vi "Kinect_Data_Detection.vi"(0 "KinectSensor References in":T1, 5 "Image":T2, 7 "Distance from Kinect (m)":dbl=1.03 format="%#_13g", 11 "error in (no error)":errorcluster) -> (1 "X (m)":dbl format="%#.2f", 2 "Y (m)":dbl format="%#.2f", 3 "Z (m)":dbl format="%#.2f", 4 "KinectSensor References":T1, 6 "Image Out":T2, 8 "Distance from Kinect (calibrated, m)":dbl, 15 "Error Out":errorcluster)   [LabVIEW 2015]
uses:
  <vilib>/MakerHub/KinectOne/Private/Type Defs/KinectSensor References.ctl
  Microsoft.Kinect
  C:/Program Files (x86)/National Instruments/LabVIEW 2015/vi.lib/MakerHub/KinectOne/Private/Libs/BodyFrameDataInterface.dll
  Program Files (x86)/National Instruments/LabVIEW 2015/vi.lib/MakerHub/KinectOne/Private/Libs/BodyFrameDataInterface.dll
  <vilib>/vision/Image Controls.llb/IMAQ Image.ctl
  <vilib>/MakerHub/KinectOne/Private/Type Defs/Joint Position.ctl
  <vilib>/MakerHub/KinectOne/Private/Type Defs/JointType.ctl
  <vilib>/MakerHub/KinectOne/Private/kinectRead [BodyFrame].vi
  <vilib>/MakerHub/KinectOne/KinectOne.lvlib
  <vilib>/ptbypt/NI_PtbyPt.lvlib
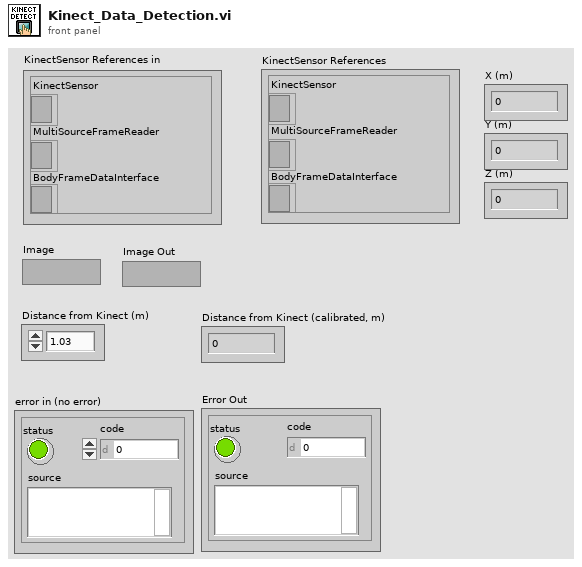
[diagram p1: front panel]
types:
  T1 = typedef "KinectOne.lvlib/KinectSensor References.ctl" = cluster{"KinectSensor":refnum<k24>, "MultiSourceFrameReader":refnum<k24>, "BodyFrameDataInterface":refnum<k24>}
  T2 = typedef "IMAQ Image.ctl" = refnum<image>
  T3 = typedef "KinectOne.lvlib/BodyData.ctl" = cluster{"ClippedEdges":T4, "HandLeftConfidence":T5, "HandLeftState":T6, "HandRightConfidence":T7, "HandRightState":T8, "IsRestricted":bool, "IsTracked":bool, "JointOrientations":refnum<k24>, "Joints":refnum<k24>, "Lean":refnum<k24>, "LeanTrackingState":T9, "TrackingId":u64}
  T4 = typedef "KinectOne.lvlib/ClippedEdges.ctl" = enum16{"None", "Right", "Left", "Top", "Bottom"}
  T5 = typedef "KinectOne.lvlib/HandLeftConfidence.ctl" = enum16{"Low", "High"}
  T6 = typedef "KinectOne.lvlib/HandLeftState.ctl" = enum16{"Unknown", "NotTracked", "Open", "Closed", "Lasso"}
  T7 = typedef "KinectOne.lvlib/HandRightConfidence.ctl" = enum16{"Low", "High"}
  T8 = typedef "KinectOne.lvlib/HandRightState.ctl" = enum16{"Unknown", "NotTracked", "Open", "Closed", "Lasso"}
  T9 = typedef "KinectOne.lvlib/LeanTrackingState.ctl" = enum16{"NotTracked", "Inferred", "Tracked"}
  T10 = typedef "KinectOne.lvlib/Joint Position.ctl" = cluster{"Camera Space":cluster{"X":dbl, "Y":dbl, "Z":dbl}, "Color Space":cluster{"X":dbl, "Y":dbl}, "Depth Space":cluster{"X":dbl, "Y":dbl}, "Tracking State":enum16{"NotTracked", "Inferred", "Tracked"}}
  T11 = typedef "KinectOne.lvlib/JointType.ctl" = enum16{"SpineBase", "SpineMid", "Neck", "Head", "ShoulderLeft", "ElbowLeft", "WristLeft", "HandLeft", "ShoulderRight", "ElbowRight", "WristRight", "HandRight", "HipLeft", "KneeLeft", "AnkleLeft", "FootLeft", "HipRight", "KneeRight", "AnkleRight", "FootRight", "SpineShoulder", "HandTipLeft", "ThumbLeft", "HandTipRight", "ThumbRight"}
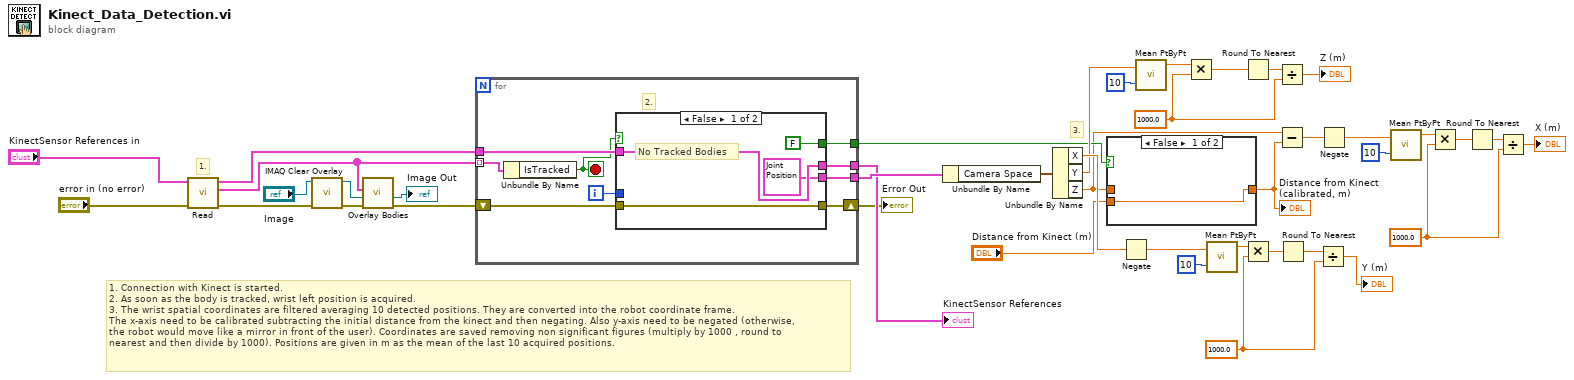
[diagram p0: block diagram]
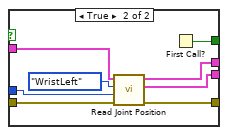
[diagram p3: hidden frame]
diagram:
  w3 = 1000.0 ("y")
  w8 = 1000.0 ("y")
  w12 = 1000.0 ("y")
  # "3."
  # "1."
  # "1. Connection with Kinect is started.\n2. As soon as the body is tracked, wrist left position is acquired.\n3. The wrist spatial coordinates are filtered averaging 10 detected positions. They are converted into the robot coordinate frame.\nThe x-axis need to be calibrated subtracting the initial distance from the kinect and then negating. Also y-axis need to be negated (otherwise,\nthe robot would move like a mirror in front of the user). Coordinates are saved removing non significant figures (multiply by 1000 , round to \nnearest and then divide by 1000). Positions are given in m as the mean of the last 10 acquired positions."
  n1 = call-poly <vilib>:"Read.vi"("error in (no error)"="error in (no error)", "KinectSensor References in"="KinectSensor References in") -> ("error out"=w41:errorcluster, "Body Data"=w38:T3[], "KinectSensor References out"=w37:T1)  [unwired: 7 in]
  n2 = call "IMAQ Clear Overlay"("error in (no error)"=w41, "Image"="Image") -> ("error out"=w39:errorcluster, "Image Out"=w40:T2)  [unwired: 8 in]
  n3 = call <vilib>:"Overlay Bodies.vi"("Error In"=w39, "Image"=w40, "Body Data"=w38) -> ("Error Out"=w36:errorcluster, "Image Out"=→"Image Out":T2)  [unwired: 7 in]
  n4 = for {
    tunnel: [w48] -> w27
    tunnel: w37 -> [w47]
    tunnel: [w46] -> w35
    shift-right: [w49] -> w26
    shift-left: w36 -> [w50]
    tunnel: w38 -> [w45] mode=indexing
    tunnel: [w42] -> w17
    i -> [w43]
    stop <- w44 stop-if-true
    # "2."
    n5 = Unbundle By Name(w45) -> ("IsTracked"=w44:bool)
    n6 = case shown="False" w44 {
      tunnel: w50 -> [w53 w62]
      tunnel: [w53 w61] -> w49
      tunnel: [w54 w60] -> w48
      tunnel: w47 -> [w54 w59]
      tunnel: [T10 {"Camera Space"={"X"=0.0, "Y"=0.0, "Z"=0.0}, "Color Space"={"X"=0.0, "Y"=0.0}, "Depth Space"={"X"=0.0, "Y"=0.0}, "Tracking State"=enum."NotTracked"} ("Joint Position") w57] -> w46
      tunnel: w43 -> [_ w56]
      tunnel: [FALSE w55] -> w42
      frame False {
        # "No Tracked Bodies"
      }
      frame True {
        n7 = call <vilib>:"Read Joint Position.vi"("Error In"=w62, "Body Index"=w56, "JointType"=JointType."WristLeft", "KinectSensor References"=w59) -> ("Error Out"=w61:errorcluster, "Joint Position"=w57:T10, "KinectSensor References"=w60:T1)  [unwired: 4 in, 1 out]
        n8 = First Call?() -> (First Call?: T/F=w55:bool)
      }
    }
  }
  "KinectSensor References" <- w27
  "Error Out" <- w26
  n9 = Unbundle By Name(w35) -> ("Camera Space"=w34:cluster{"X":dbl, "Y":dbl, "Z":dbl})
  n10 = Unbundle By Name(w34) -> ("X"=w33:dbl, "Y"=w20:dbl, "Z"=w16:dbl)
  n11 = case shown="False" w17 {
    tunnel: "Distance from Kinect (m)" -> [w63 _]
    tunnel: [w63 w64] -> w18
    tunnel: w16 -> [_ w64]
    frame False {
    }
    frame True {
    }
  }
  "Distance from Kinect (calibrated, m)" <- w18
  n12 = Negate(x=w33) -> (-x=w22:dbl)
  n13 = call <vilib>:"Mean PtByPt.vi"("x"=w20, "sample length"=10) -> ("mean"=w2:dbl)  [unwired: 2 in, 1 out]
  n14 = Multiply(x=w2, y=w3) -> (x*y=w5:dbl)
  n15 = call <vilib>:"Mean PtByPt.vi"("x"=w22, "sample length"=10) -> ("mean"=w15:dbl)  [unwired: 2 in, 1 out]
  n16 = Round To Nearest(number=w5) -> (nearest integer value=w4:dbl)
  n17 = Multiply(x=w15, y=w12) -> (x*y=w14:dbl)
  n18 = Divide(x=w4, y=w3) -> (x/y=→"Z (m)":dbl)
  n19 = Subtract(x=w16, y=w18) -> (x-y=w32:dbl)
  n20 = Round To Nearest(number=w14) -> (nearest integer value=w13:dbl)
  n21 = Divide(x=w13, y=w12) -> (x/y=→"Y (m)":dbl)
  n22 = Negate(x=w32) -> (-x=w25:dbl)
  n23 = call <vilib>:"Mean PtByPt.vi"("x"=w25, "sample length"=10) -> ("mean"=w7:dbl)  [unwired: 2 in, 1 out]
  n24 = Multiply(x=w7, y=w8) -> (x*y=w10:dbl)
  n25 = Round To Nearest(number=w10) -> (nearest integer value=w9:dbl)
  n26 = Divide(x=w9, y=w8) -> (x/y=→"X (m)":dbl)
